vi "BT Rx Test Get BT INSTR TX.vi"(8 "error in (no error)":errorcluster, 11 "niDTS BT Rx Test in":refnum<class "niDTS BT Rx Test.lvclass">) -> (0 "error out":errorcluster, 2 "niDTS BT.lvlib:niDTS BT INSTR RX":refnum<class "niDTS BT INSTR RX.lvclass">, 3 "niDTS BT Rx Test out":refnum<class "niDTS BT Rx Test.lvclass">)   [LabVIEW 2015, in "niDTS BT.lvlib" / "niDTS BT Rx Test.lvclass"]
uses:
  niDTS BT Rx Test.lvclass
  Instrument/INSTR RX/niDTS BT INSTR RX.lvclass
  niDTS BT Rx Test.lvclass/niDTS BT Rx Test.ctl
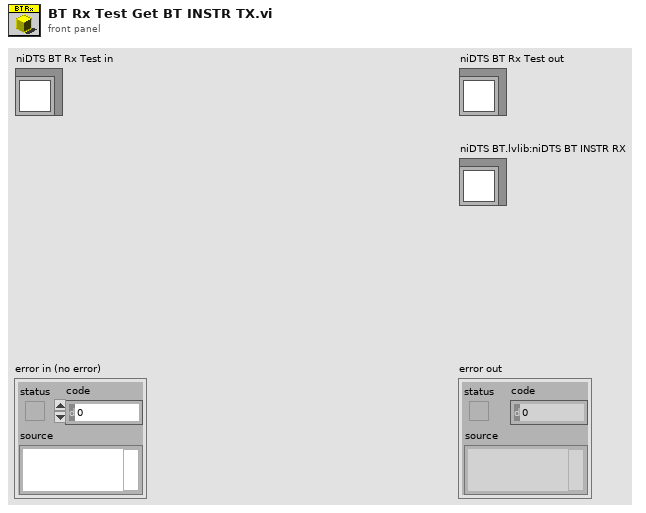
[diagram p1: front panel]
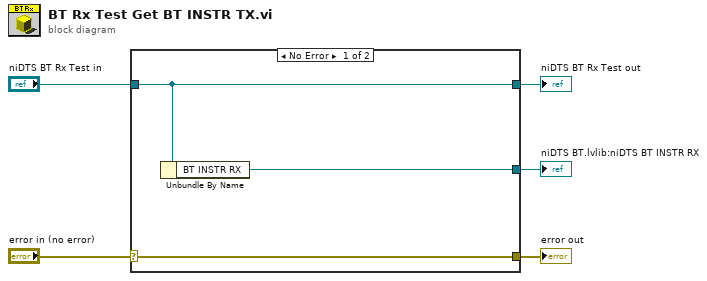
[diagram p0: block diagram]
diagram:
  n1 = case shown="No Error" "error in (no error)" {
    selector: "error in (no error)" -> [w8 w9]
    tunnel: [w8 w9] -> w4
    tunnel: [w7 w10] -> w2
    tunnel: "niDTS BT Rx Test in" -> [w7 w10]
    tunnel: [w6 _] -> w1
    frame No Error {
      n2 = Unbundle By Name(w7) -> ("BT INSTR RX"=w6:refnum<class "niDTS BT INSTR RX.lvclass">)
    }
    frame Error {
    }
  }
  "error out" <- w4
  "niDTS BT Rx Test out" <- w2
  "niDTS BT.lvlib:niDTS BT INSTR RX" <- w1
